vi "mask picture.vi"(9 "mask color":u32(colorbox)=6618880, 11 "new picture in":picture) -> (3 "new picture out":picture)   [LabVIEW 2023]
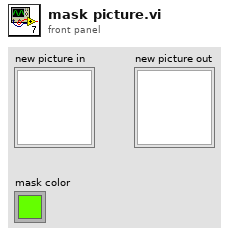
[diagram p1: front panel]
types:
  T1 = typedef "imagedata.ctl" = cluster{"image type":i32, "image depth":i32, "image":u8[], "mask":u8[], "colors":u32[], "Rectangle":cluster{"left":i16, "top":i16, "right":i16, "bottom":i16}}
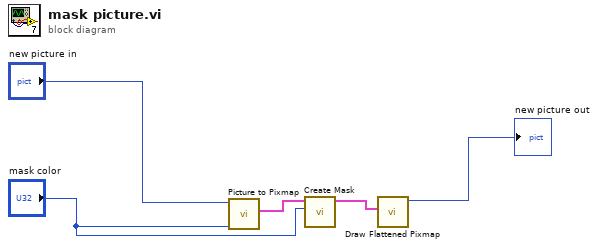
[diagram p0: block diagram]
diagram:
  n1 = call <vilib>:"Picture to Pixmap.vi"("Background Color"="mask color", "picture"="new picture in") -> ("image data"=w3:T1)  [unwired: 8 in, 1 out]
  n2 = call <vilib>:"Create Mask.vi"("Mask Color (Black)"="mask color", "image data"=w3) -> ("image data"=w4:T1)  [unwired: 9 in]
  n3 = call <vilib>:"Draw Flattened Pixmap.vi"("image data"=w4) -> ("new picture"=→"new picture out":picture)  [unwired: 8 in]
